vi "Capture@LoadNextImaq__Parameter.vi"(1 "ParamterIn":string) -> (0 "ParamterOut":string)   [LabVIEW 2019]
panel:
  in  "IMAQName":string(combo)
  in  "CamName":string(combo)
  in  "Confirm":bool
  # "Capture@LoadImaqNex $Capture(,$ImaqName)"
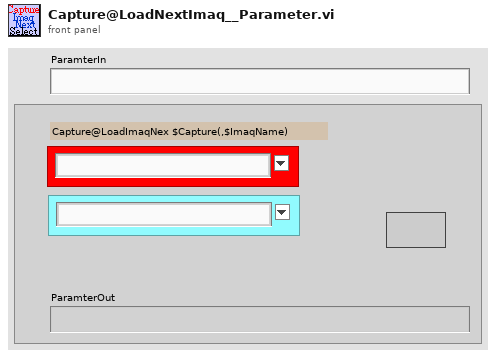
[diagram p1: front panel]
types:
  T1 = enum16{"Get", "Get&Index+1", "Insert", "Init", "Clear", "SetIndex"}
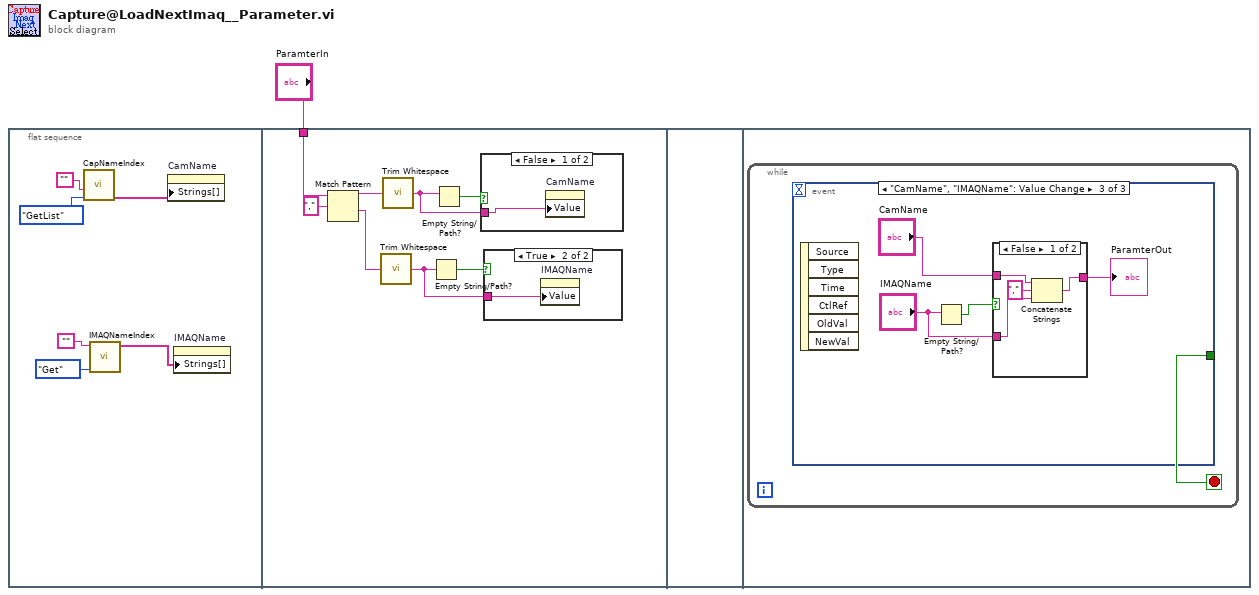
[diagram p0: block diagram]
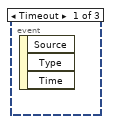
[diagram p4: hidden frame]
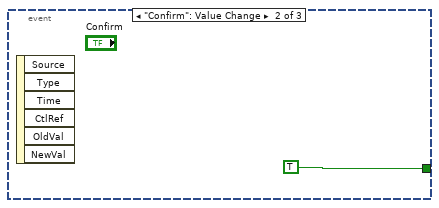
[diagram p5: hidden frame]
diagram:
  n1 = flat-sequence {
    tunnel: "ParamterIn" -> [w14]
    frame #0 {
      n2 = call "CapNameIndex.vi"("OP"=enum16{"AddCam", "GetIndex", "Init", "GetList"}."GetList", "CamName"="") -> ("DeviceList"=w6:string[])  [unwired: 2 in, 3 out]
      n3 = call "IMAQNameIndex.vi"("OP"=T1."Get", "IMAQName"="") -> ("IMAQNameList"=w2:string[])  [unwired: 2 in, 7 out]
      n4 = property on="CamName" class="CmbBox"("Strings[]"=w6) -> ()  [unwired: 2 in, 2 out]
      n5 = property on="IMAQName" class="CmbBox"("Strings[]"=w2) -> ()  [unwired: 2 in, 2 out]
    }
    frame #1 {
      n6 = Match Pattern(string=w14, regular expression=",") -> (before substring=w11:string, after substring=w10:string)  [unwired: 1 in, 2 out]
      n7 = call <vilib>:"Trim Whitespace.vi"("string"=w10) -> ("trimmed string"=w8:string)  [unwired: 1 in]
      n8 = call <vilib>:"Trim Whitespace.vi"("string"=w11) -> ("trimmed string"=w12:string)  [unwired: 1 in]
      n9 = Empty String/Path?(string/path=w8) -> (empty?=w9:bool)
      n10 = Empty String/Path?(string/path=w12) -> (empty?=w15:bool)
      n11 = case shown="False" w15 {
        tunnel: w12 -> [w17 _]
        frame False {
          n12 = property on="CamName" class="CmbBox"("Value"=w17) -> ()  [unwired: 2 in, 2 out]
        }
        frame True {
        }
      }
      n13 = case shown="True" w9 {
        tunnel: w8 -> [_ w16]
        frame False {
        }
        frame True {
          n14 = property on="IMAQName" class="CmbBox"("Value"=w16) -> ()  [unwired: 2 in, 2 out]
        }
      }
    }
    frame #2 {
    }
    frame #3 {
      n15 = while {
        stop <- w18 stop-if-true
        n16 = event shown="[2] \"CamName\", \"IMAQName\": Value Change" {
          selector: _ -> [_ _ _]
          dyn-events: _ -> [_ _ _]
          timeout: _ -> [_ _ _]
          tunnel: [_ TRUE _] -> w18
          event Timeout {
            n17 = event-data() -> ()  [unwired: 1 in, 3 out]
          }
          event "Confirm": Value Change {
            n18 = event-data() -> ()  [unwired: 1 in, 6 out]
          }
          event "CamName", "IMAQName": Value Change {
            n19 = event-data() -> ()  [unwired: 1 in, 6 out]
            n20 = Empty String/Path?(string/path="IMAQName") -> (empty?=w23:bool)
            n21 = case shown="False" w23 {
              tunnel: [w24 w28] -> w21
              tunnel: "CamName" -> [w27 w28]
              tunnel: "IMAQName" -> [w26 _]
              frame False {
                n22 = Concatenate Strings(w27, "," ("string"), w26) -> (w24:string)
              }
              frame True {
              }
            }
            "ParamterOut" <- w21
          }
        }
      }
    }
  }
